vi "Update Trigger Status.vi"(8 "error in (no error)":errorcluster, 9 "Ready for Trigger":bool, 10 "Camera ID":i32, 11 "Virtual Camera in":refnum<class "Virtual Camera.lvclass">) -> (0 "error out":errorcluster, 3 "Virtual Camera out":refnum<class "Virtual Camera.lvclass">)   [LabVIEW 2015]
uses:
  Virtual Camera.lvclass
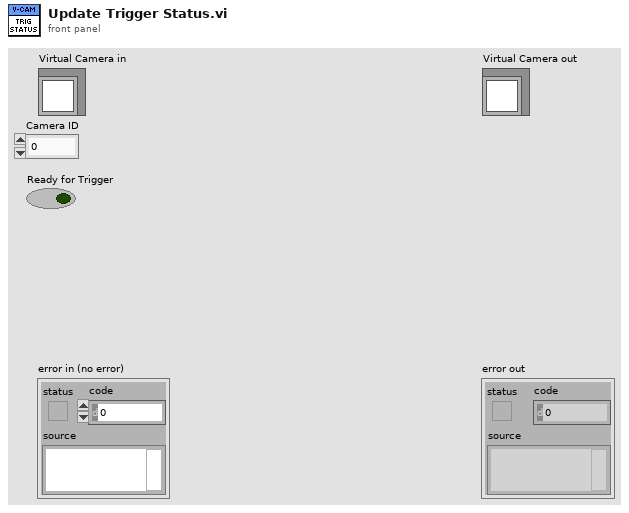
[diagram p1: front panel]
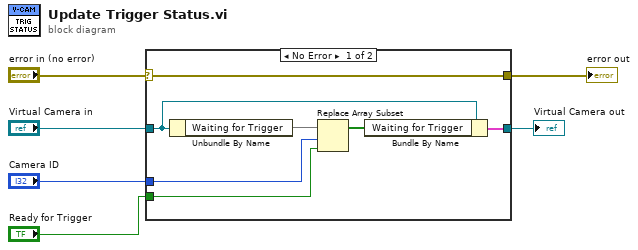
[diagram p0: block diagram]
diagram:
  n1 = case shown="No Error" "error in (no error)" {
    selector: "error in (no error)" -> [w13 w15]
    tunnel: [w13 w15] -> w5
    tunnel: [w8 w14] -> w3
    tunnel: "Virtual Camera in" -> [w9 w14]
    tunnel: "Camera ID" -> [w12 _]
    tunnel: "Ready for Trigger" -> [w10 _]
    frame No Error {
      n2 = Unbundle By Name(w9) -> ("Waiting for Trigger"=w7)
      n3 = Replace Array Subset(array=w7, new element=w10, index=w12) -> (w11:bool[])
      n4 = Bundle By Name(cluster=w9, "Waiting for Trigger"=w11) -> (w8:cluster{})
    }
    frame Error {
    }
  }
  "error out" <- w5
  "Virtual Camera out" <- w3
